vi "Controller_2_2_Proportional.vi"() -> ()   [LabVIEW 2019]
uses:
  <vilib>/myRIO/Instrument Drivers/Onboard IO/AI/typedefs/AI Reference.ctl
  <vilib>/myRIO/Common/Instrument Driver Framework/Utilities/typedefs/myRIO Generic Hardware Reference.ctl
  <vilib>/myRIO/Common/Instrument Driver Framework/Utilities/typedefs/Hardware Version Enum.ctl
  <vilib>/myRIO/Common/Instrument Driver Framework/Utilities/typedefs/myRIO v1.0 Reference.ctl
  <vilib>/myRIO/Common/Instrument Driver Framework/Utilities/typedefs/Generic FPGA Reference.ctl
  <vilib>/myRIO/Common/Instrument Driver Framework/myRIO v1.0/AI/typedefs/AI Channels List.ctl
  <vilib>/myRIO/Common/Instrument Driver Framework/myRIO v1.0/AI/typedefs/AI Channels Enum.ctl
  <vilib>/myRIO/Common/Instrument Driver Framework/Utilities/typedefs/Analog Scaling Constants List.ctl
  <vilib>/myRIO/Common/Instrument Driver Framework/Utilities/typedefs/Analog Scaling Constants.ctl
  <vilib>/userDefined/High Color/nirio_resource_hc.ctl
  <vilib>/myRIO/Instrument Drivers/Onboard IO/PWM/typedefs/PWM Reference.ctl
  <vilib>/myRIO/Common/Instrument Driver Framework/myRIO v1.0/PWM/typedefs/PWM Channels Enum.ctl
  <vilib>/myRIO/Instrument Drivers/Onboard IO/PWM/typedefs/PWM Configuration.ctl
  <vilib>/myRIO/Common/Instrument Driver Framework/Utilities/vis/Is FPGA Ref Available.vi
  <vilib>/myRIO/Common/Instrument Driver Framework/myRIO v1.0/AI/vis/myRIO v1.1 Open AI.vi
  <vilib>/myRIO/Instrument Drivers/Onboard IO/AI/vis/Read.vi
  <vilib>/myRIO/Common/Instrument Driver Framework/myRIO v1.0/PWM/vis/myRIO v1.1 Open PWM.vi
  <vilib>/myRIO/Instrument Drivers/Onboard IO/PWM/vis/Set Duty Cycle and Frequency.vi
  <vilib>/myRIO/Common/Instrument Driver Framework/Utilities/vis/Validate Channels.vi
  <vilib>/myRIO/Common/Instrument Driver Framework/myRIO v1.0/AI/vis/myRIO v1.0 Reserve AI.vi
  <vilib>/myRIO/Common/Instrument Driver Framework/myRIO v1.0/PWM/vis/myRIO v1.0 Reserve PWM.vi
  <vilib>/myRIO/Common/Instrument Driver Framework/myRIO v1.0/UART/vis/myRIO v1.0 Close UART.vi
  <vilib>/myRIO/Common/Instrument Driver Framework/myRIO v1.0/AI/vis/myRIO v1.0 Build MUX Configuration AI.vi
  <vilib>/myRIO/Common/Instrument Driver Framework/myRIO v1.0/Resource Manager/vis/myRIO v1.0 Reserve Channel List.vi
  <vilib>/myRIO/Common/Instrument Driver Framework/myRIO v1.0/PWM/vis/myRIO v1.0 Build MUX Configuration PWM.vi
  <vilib>/myRIO/Common/Instrument Driver Framework/myRIO v1.0/Resource Manager/vis/myRIO v1.0 Reserve Channel.vi
  <vilib>/myRIO/Common/Instrument Driver Framework/myRIO v1.0/Resource Manager/vis/myRIO v1.0 Unreserve Channel.vi
  <vilib>/myRIO/Common/Instrument Driver Framework/myRIO v1.0/Resource Manager/vis/myRIO v1.0 Create Configuration List.vi
  <vilib>/myRIO/Common/Instrument Driver Framework/myRIO v1.0/Resource Manager/vis/myRIO v1.0 Build Mutex Name.vi
  <vilib>/Utility/VariantDataType/GetNumericInfo.vi
  <vilib>/Utility/error.llb/Error Cluster From Error Code.vi
  <vilib>/myRIO/Common/Instrument Driver Framework/myRIO v1.0/myRIO v1.1 Open.vi
  <vilib>/myRIO/Common/Instrument Driver Framework/myRIO v1.0/AI/vis/myRIO v1.0 Get Scaling Constants AI.vi
  <vilib>/myRIO/Common/Instrument Driver Framework/Utilities/vis/IO Manager.vi
  <vilib>/myRIO/Common/Instrument Driver Framework/Utilities/vis/Configuration Manager.vi
  <vilib>/myRIO/Common/Instrument Driver Framework/myRIO v1.0/myRIO v1.0 Close.vi
  <vilib>/myRIO/Common/Instrument Driver Framework/myRIO v1.0/AI/vis/myRIO v1.0 Read AI.vi
  <vilib>/imath/engines/lvmath2/RunTimeEngine/Managers/WorkSpace/UID Generator.vi
  <vilib>/imath/engines/lvmath2/RunTimeEngine/RunTimeType/NIMS_RunTimeType_From StrictType (excl LVString).vi
  <instcachedir>/0/NIMS_RunTimeType_From StrictType (excl LVString)_D8AFBA86A94845AAA577C895450664BD.lvgen/NIMS_RunTimeType_From StrictType (excl LVString)_D8AFBA86A94845AAA577C895450664BD_000.vi
  <vilib>/imath/engines/lvmath2/RunTimeEngine/LocalVariableDefStatement/MC_LocalVariableDefStatement_Display.vi
  <vilib>/imath/engines/lvmath2/RunTimeEngine/Managers/SymbolTable/Clear UID.vi
  <vilib>/imath/engines/lvmath2/RunTimeEngine/NodeEndStatement/NIMS_NodeEndStatement_Output.vi
  <instcachedir>/0/NIMS_NodeEndStatement_Output_53EC0D466D134D7ABD903AC30B43404B.lvgen/NIMS_NodeEndStatement_Output_53EC0D466D134D7ABD903AC30B43404B_001.vi
  <vilib>/imath/engines/lvmath2/RunTimeEngine/ErrorHandling/NIMS_Finalize Error.vi
  <vilib>/myRIO/Common/Instrument Driver Framework/myRIO v1.0/Resource Manager/vis/myRIO v1.0 Configure IO.vi
  <vilib>/myRIO/Common/Instrument Driver Framework/myRIO v1.0/PWM/vis/myRIO v1.0 Write PWM.vi
  <vilib>/addons/control/pid/pid.llb/PID (DBL).vi
  <vilib>/myRIO/Common/Instrument Driver Framework/Utilities/vis/FPGA Ref Manager.vi
  <vilib>/myRIO/Common/Instrument Driver Framework/myRIO v1.0/myRIO v1.0 Reset FPGA.vi
  <vilib>/myRIO/Common/Instrument Driver Framework/myRIO v1.0/IRQ/vis/myRIO v1.0 IRQ Info FGV.vi
  <vilib>/myRIO/Common/Instrument Driver Framework/myRIO v1.0/IRQ/vis/myRIO v1.0 Timer IRQ Info FGV.vi
  <vilib>/myRIO/Common/Instrument Driver Framework/myRIO v1.0/IRQ/vis/myRIO v1.0 ISR Agent.vi
  <vilib>/myRIO/Instrument Drivers/Utilities/vis/Reset Index.vi
  <vilib>/myRIO/Common/Instrument Driver Framework/myRIO v1.0/Resource Manager/vis/myRIO v1.0 Block Write Resource Manager.vi
  <vilib>/myRIO/Express VI/Onboard IO/AI/AI Express VI.xnode
  <vilib>/myRIO/Instrument Drivers/Onboard IO/AI/vis/myRIO AI Open.xnode
  <vilib>/myRIO/Express VI/Onboard IO/PWM/PWM Express VI.xnode
  <vilib>/myRIO/Instrument Drivers/Onboard IO/PWM/vis/myRIO PWM Open.xnode
  <vilib>/myRIO/Instrument Drivers/Onboard IO/PWM/PWM.lvlib
  <vilib>/myRIO/Instrument Drivers/Onboard IO/AI/AI.lvlib
  <vilib>/imath/engines/lvmath2/RunTimeEngine/Managers/SymbolTable/NIMS_WorkSpace.lvlib
  <vilib>/addons/control/pid/NI_PID_pid.lvlib
  <vilib>/ptbypt/NI_PtbyPt.lvlib
  <vilib>/myRIO/Instrument Drivers/Utilities/Utilities.lvlib
panel:
  out "Duty Cycle":dynamicdata(graph)
  out "Pressure Actuator":dynamicdata(graph)
  out "Pressures Actuator":cluster{dbl, dbl}(knob)={0.0, 8.870406975580165} scale=0.0..120.0
  in  "stop":bool
  out "VA_sensor":dbl format="%#.3g"
  out "Pressures Receiver":cluster{dbl, dbl}(knob)={0.0, 8.870406975580165} scale=0.0..120.0
  in  "Setpoint Preceiver":dbl(slide) scale=0.0..80.0
  out "V_Rsensor":dbl format="%#.3g"
  in  "PID Motor":T1={"proportional gain (Kc)"=0.01, "integral time (Ti, min)"=0.005, "derivative time (Td, min)"=0.0} {"derivative time (Td, min)" format="%.3f"; "integral time (Ti, min)" format="%.3f"; "proportional gain (Kc)" format="%.3f"}
  out "Duty cycle Motor":dbl(knob) scale=0.0..1.0
  in  "Setpoint Pactuator":dbl(slide) scale=0.0..70.0
  in  "milliseconds to wait":u32=100
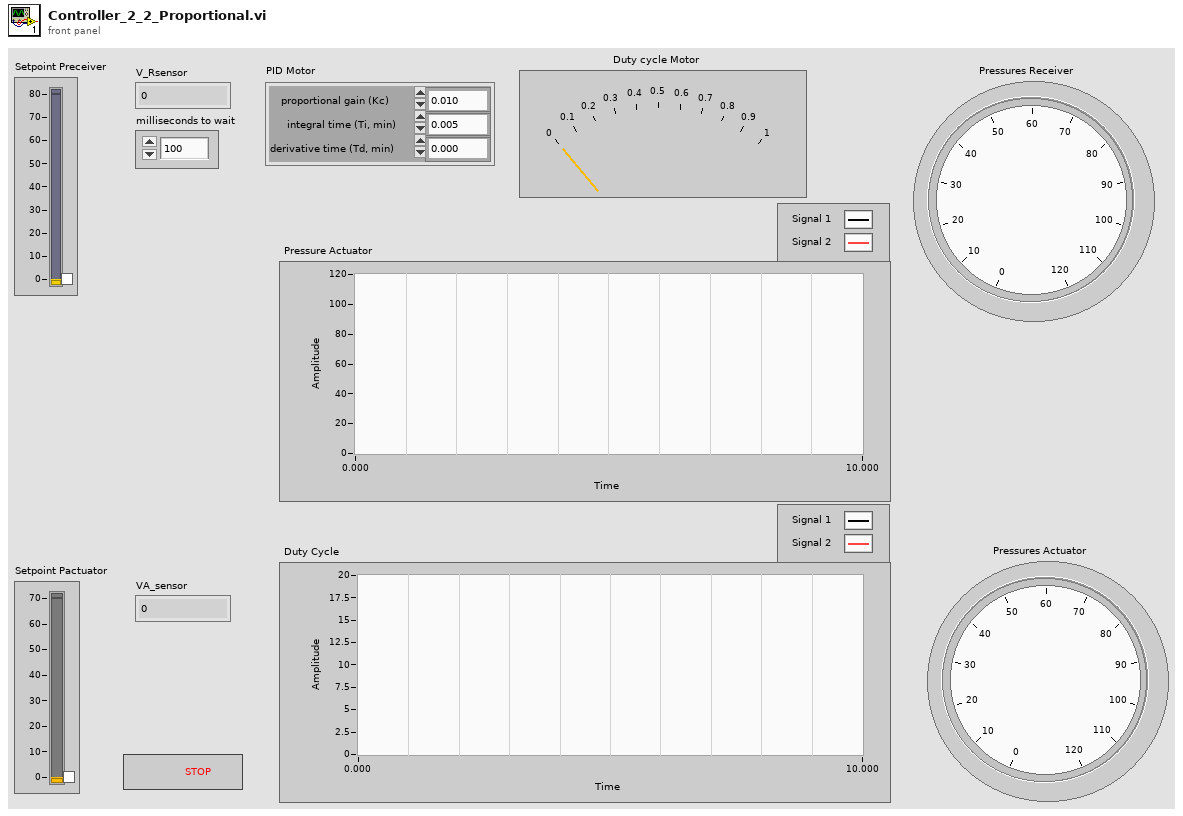
[diagram p1: front panel]
types:
  T1 = cluster{"proportional gain (Kc)":dbl, "integral time (Ti, min)":dbl, "derivative time (Td, min)":dbl}
  T2 = typedef "PWM.lvlib/PWM Reference.ctl" = cluster{"myRIO Reference":T3, "PWM Channels Enum":T7, "PWM Configuration":T8}
  T3 = typedef "myRIO Generic Hardware Reference.ctl" = cluster{"myRIO Model":T4, "myRIO Hardware Reference":T5}
  T4 = typedef "Hardware Version Enum.ctl" = enum16{"Unknown", "myRIO-1900", "myRIO-1950", "roboRIO", "NI ELVIS RIO CM", "ELVIS III"}
  T5 = typedef "myRIO v1.0 Reference.ctl" = cluster{"Generic FPGA Reference":T6, "Allow multiple opens":bool}
  T6 = typedef "Generic FPGA Reference.ctl" = refnum<k20>
  T7 = typedef "PWM Channels Enum.ctl" = enum16{"Not Connected", "C/PWM0", "C/PWM1", "A/PWM0", "A/PWM1", "A/PWM2", "A/PWM3", "A/PWM4", "A/PWM5", "A/PWM6", "A/PWM7", "A/PWM8", "A/PWM9", "A/PWM10", "A/PWM11", "A/PWM12", "A/PWM13", "A/PWM14", "A/PWM15", "A/PWM16", "A/PWM17", "A/PWM18", "A/PWM19", "B/PWM0", "B/PWM1", "B/PWM2", "B/PWM3", "B/PWM4", "B/PWM5", "B/PWM6", "B/PWM7", "B/PWM8", "B/PWM9", "B/PWM10", "B/PWM11", "B/PWM12", "B/PWM13", "B/PWM14", "B/PWM15", "B/PWM16", "B/PWM17", "B/PWM18", "B/PWM19", "PWM/PWM0", "PWM/PWM1", "PWM/PWM2", "PWM/PWM3", "PWM/PWM4", "PWM/PWM5", "PWM/PWM6", "PWM/PWM7", "PWM/PWM8", "PWM/PWM9"}
  T8 = typedef "PWM.lvlib/PWM Configuration.ctl" = cluster{"Frequency":dbl, "Duty Cycle":dbl}
  T9 = typedef "nirio_resource_hc.ctl" = tag
  T10 = typedef "AI.lvlib/AI Reference.ctl" = cluster{"myRIO Reference":T3, "AI Channels List":T11, "AI Scaling Constants List":T13}
  T11 = typedef "AI Channels List.ctl" = T12[]
  T12 = typedef "AI Channels Enum.ctl" = enum16{"Not Connected", "AudioIn/Left", "AudioIn/Right", "C/AI0", "C/AI1", "A/AI0", "A/AI1", "A/AI2", "A/AI3", "A/AI4", "A/AI5", "A/AI6", "A/AI7", "B/AI0", "B/AI1", "B/AI2", "B/AI3", "B/AI4", "B/AI5", "B/AI6", "B/AI7", "AI/AI0", "AI/AI1", "AI/AI2", "AI/AI3", "A/AI0 (DIFF)", "A/AI1 (DIFF)", "A/AI2 (DIFF)", "A/AI3 (DIFF)", "B/AI0 (DIFF)", "B/AI1 (DIFF)", "B/AI2 (DIFF)", "B/AI3 (DIFF)"}
  T13 = typedef "Analog Scaling Constants List.ctl" = T14[]
  T14 = typedef "Analog Scaling Constants.ctl" = cluster{"LSB Weight (Volts)":dbl, "Offset (Volts)":dbl, "Signed?":bool}
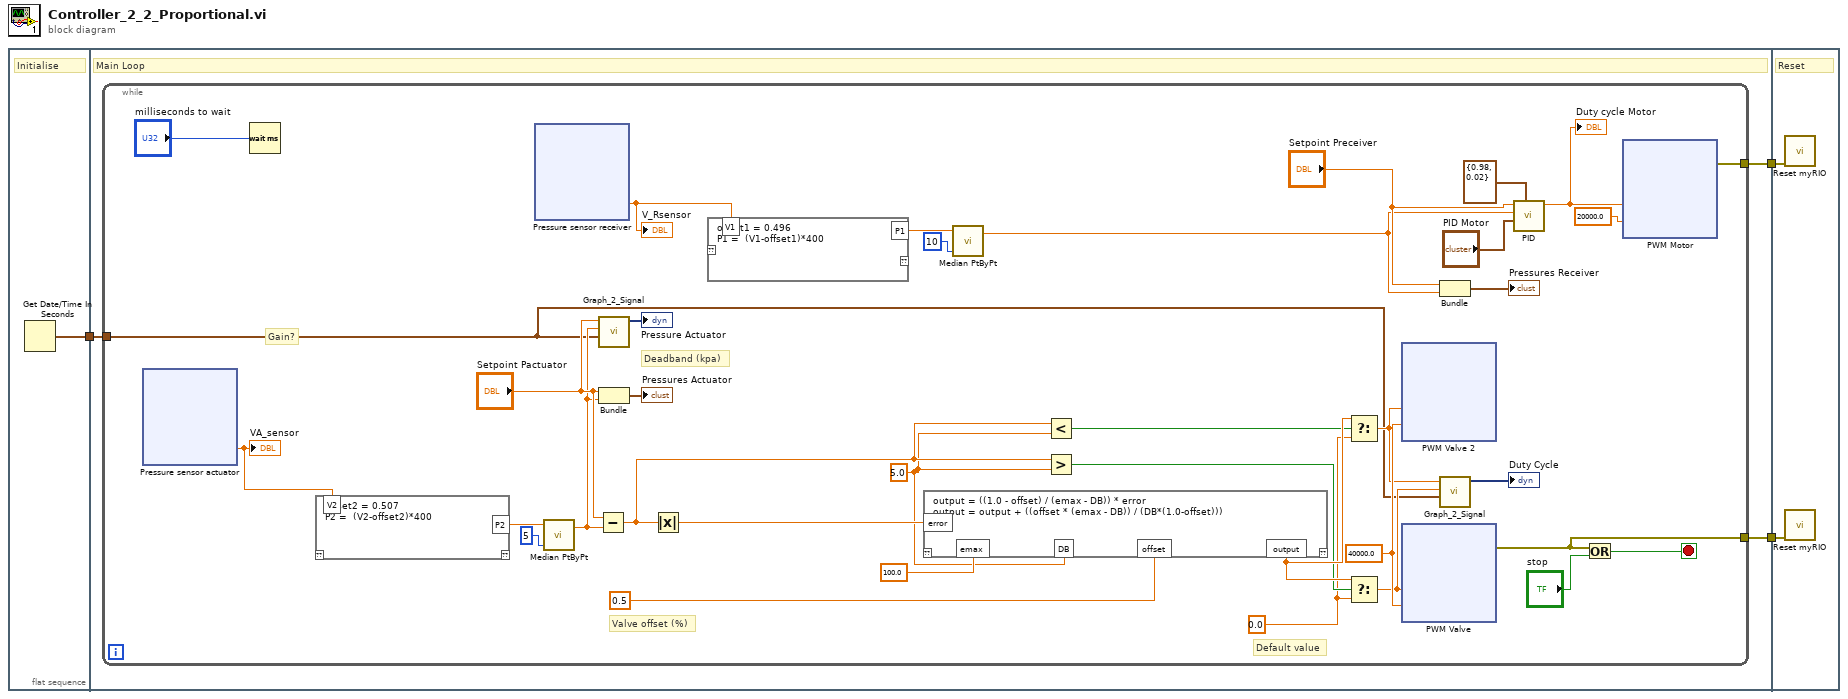
[diagram p0: block diagram]
diagram:
  n1 = flat-sequence {
    tunnel: [w4] -> w3
    tunnel: [w7] -> w2
    tunnel: [w6] -> w1
    tunnel: w3 -> [w5]
    tunnel: w2 -> [w397]
    tunnel: w1 -> [w396]
    frame #0 {
      # "Initialise"
      n2 = Get Date/Time In Seconds() -> (seconds since 1Jan1904=w4:timestamp)
    }
    frame #1 {
      # "Main Loop"
      n3 = while {
        tunnel: [w42] -> w7
        tunnel: [w29] -> w6
        tunnel: w5 -> [w8]
        stop <- w41 stop-if-true
        w16 = 5.0 ("Frequency [Hz]")
        w19 = 0.0 ("Frequency [Hz]")
        w25 = 40000.0 ("Frequency [Hz]")
        # "Valve offset (%)"
        # "Deadband (kpa)"
        # "Gain?"
        # "Default value"
        n4 = xnode "Pressure sensor actuator"() -> ("A/AI0 (Pin 3)"=w40:dbl)  [unwired: 1 in, 1 out]
        "VA_sensor" <- w40
        n5 = Wait (ms)(milliseconds to wait="milliseconds to wait") -> ()  [unwired: 1 out]
        n6 = mathscript code="offset2 = 0.507\nP2 =  (V2-offset2)*400"("V2"=w40) -> ("P2"=w39:dbl)  [unwired: 1 in, 1 out]
        n7 = xnode "Pressure sensor receiver"() -> ("A/AI1 (Pin 5)"=w28:dbl)  [unwired: 1 in, 1 out]
        "V_Rsensor" <- w28
        n8 = call <vilib>:"Median PtByPt.vi"("sample length"=5, "x"=w39) -> ("median"=w11:dbl)  [unwired: 2 in, 1 out]
        n9 = Subtract(x="Setpoint Pactuator", y=w11) -> (x-y=w24:dbl)
        n10 = call "Graph_2_Signal.vi"("y"=w8, "Dynamic Data 2"=w11, "Dynamic Data 1"="Setpoint Pactuator") -> ("Signals"=→"Pressure Actuator":dynamicdata)  [unwired: 8 in]
        n11 = Bundle("Setpoint Pactuator"="Setpoint Pactuator", "median"=w11) -> (→"Pressures Actuator":cluster{"Setpoint Pactuator":dbl, "median":dbl})  [unwired: 1 in]
        n12 = Absolute Value(x=w24) -> (abs(x)=w23:dbl)
        n13 = mathscript code="offset1 = 0.496\nP1 =  (V1-offset1)*400"("V1"=w28) -> ("P1"=w31:dbl)  [unwired: 1 in, 1 out]
        n14 = mathscript code="output = ((1.0 - offset) / (emax - DB)) * error\noutput = output + ((offset * (emax - DB)) / (DB*(1.0-offset)))"("error"=w23, "offset"=0.5 ("Frequency [Hz]"), "emax"=100.0 ("Frequency [Hz]"), "DB"=w16) -> ("output"=w22:dbl)  [unwired: 1 in, 1 out]
        n15 = call <vilib>:"Median PtByPt.vi"("sample length"=10, "x"=w31) -> ("median"=w33:dbl)  [unwired: 2 in, 1 out]
        n16 = Less?(x=w24, y=w16) -> (x < y?=w20:bool)
        n17 = Greater?(x=w24, y=w16) -> (0:w21:bool)
        n18 = Select(t=w22, s=w20, f=w19) -> (s? t:f=w14:dbl)
        n19 = Select(t=w22, s=w21, f=w19) -> (s? t:f=w13:dbl)
        n20 = xnode "PWM Valve 2"("Duty Cycle"=w14, "Frequency [Hz]"=w25) -> ()  [unwired: 1 in, 1 out]
        n21 = xnode "PWM Valve"("Duty Cycle"=w13, "Frequency [Hz]"=w25) -> ("error out"=w42:errorcluster)  [unwired: 1 in]
        n22 = Bundle("Setpoint Preceiver"="Setpoint Preceiver", "median"=w33) -> (→"Pressures Receiver":cluster{"Setpoint Preceiver":dbl, "median":dbl})  [unwired: 1 in]
        n23 = call "Graph_2_Signal.vi"("y"=w8, "Dynamic Data 2"=w13, "Dynamic Data 1"=w14) -> ("Signals"=→"Duty Cycle":dynamicdata)  [unwired: 8 in]
        n24 = call-poly <vilib>:"PID.vi"("output range"=cluster{"output high":dbl, "output low":dbl} {"output high"=0.98, "output low"=0.02} ("output range motor"), "PID gains"="PID Motor", "process variable"=w33, "setpoint"="Setpoint Preceiver") -> ("output"=w27:dbl)  [unwired: 6 in, 1 out]
        "Duty cycle Motor" <- w27
        n25 = Or(x=w42, y="stop") -> (x .or. y?=w41:bool)
        n26 = xnode "PWM Motor"("Duty Cycle"=w27, "Frequency [Hz]"=20000.0) -> ("error out"=w29:errorcluster)  [unwired: 1 in]
      }
    }
    frame #2 {
      # "Reset"
      n27 = call <vilib>:"Reset myRIO.vi"("error in (no error)"=w396) -> ()  [unwired: 10 in, 1 out]
      n28 = call <vilib>:"Reset myRIO.vi"("error in (no error)"=w397) -> ()  [unwired: 10 in, 1 out]
    }
  }
